vi "Simultaneous Sound Input Output.vi"() -> ()   [LabVIEW 2023]
doc: "This VI illustrates how to perform simultaneous sound IO, i.e., how to continuously play the sound acquired from a microphone. It requires the use of a microphone attached to the sound card. You can specify the IDs of the input and output devices, the frequency to sample at, and the buffer size for both devices. Higher frequencies have better quality, but demand more resources and are limited by the capabilities of your sound card. A large number of samples decreases the risk of glitches, but increases the delay between acquisition and playback."
uses:
  <vilib>/sound2/lvsound2.llb/Sampling Mode.ctl
  <vilib>/sound2/lvsound2.llb/Sound Data Format.ctl
  <vilib>/sound2/lvsound2.llb/Sound Output Write (DBL Single).vi
  <vilib>/sound2/lvsound2.llb/Sound Input Read (DBL).vi
  <vilib>/sound2/lvsound2.llb/Sound Output Write (DBL).vi
panel:
  out "Acquired Sound":waveform(dbl)[](graph)
  in  "Stop":bool
  in  "Input Device ID":u32
  in  "Output Device ID":u32
  # "Overview: Demonstrates the use of the Sound Functions to continuously play the sound acquired from a microphone.\nRequirements: Microphone\nInstructions:\n1. Specify the Input Device ID and the Output Device ID.\n2. Run the VI.\n3. Click Stop to stop the VI."
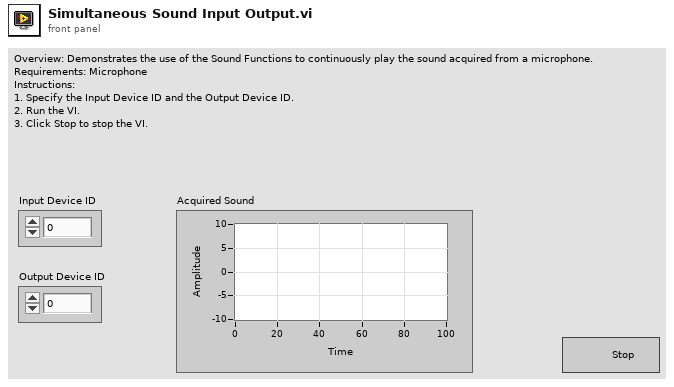
[diagram p1: front panel]
types:
  T1 = typedef "Sound Data Format.ctl" = cluster{"sample rate (S/s)":dbl, "number of channels":i32, "bits per sample":i32}
  T2 = typedef "Sampling Mode.ctl" = i32
  T3 = typedef "Sound Output Task ID.ctl" = u32
  T4 = typedef "Sound Input Task ID.ctl" = u32
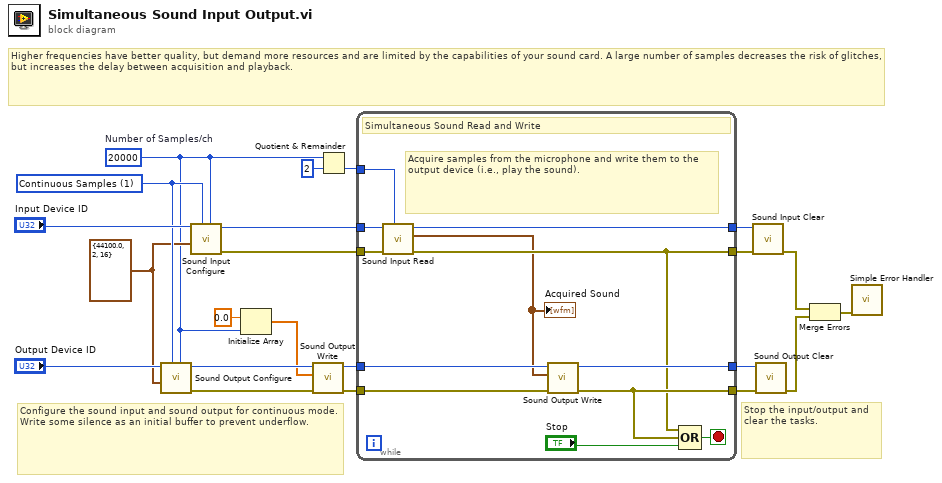
[diagram p0: block diagram]
diagram:
  w2 = 20000  # Number of Samples/ch
  w6 = T1 {"sample rate (S/s)"=44100.0, "number of channels"=2, "bits per sample"=16} ("Sound Format")
  w12 = T2 1 items=["Finite Samples", "Continuous Samples"] ("sample mode")
  # "Higher frequencies have better quality, but demand more resources and are limited by the capabilities of your sound card. A large number of samples decreases the risk of glitches, but increases the delay between acquisition and playback."
  # "Stop the input/output and clear the tasks."
  # "Configure the sound input and sound output for continuous mode. Write some silence as an initial buffer to prevent underflow."
  n1 = call <vilib>:"Sound Output Configure.vi"("number of samples/ch"=w2, "sample mode"=w12, "sound format"=w6, "device ID"="Output Device ID") -> ("error out"=w10:errorcluster, "task ID"=w11:T3)  [unwired: 6 in]
  n2 = call <vilib>:"Sound Input Configure.vi"("number of samples/ch"=w2, "sample mode"=w12, "sound format"=w6, "device ID"="Input Device ID") -> ("error out"=w14:errorcluster, "task ID"=w13:T4)  [unwired: 6 in]
  n3 = Initialize Array(0.0 ("element"), w2) -> (w4:dbl[])
  n4 = call-poly <vilib>:"Sound Output Write.vi"("error in (no error)"=w10, "data"=w4, "task ID"=w11) -> ("error out"=w9:errorcluster, "task ID out"=w8:T3)  [unwired: 7 in]
  n5 = Quotient & Remainder(x=w2, y=2) -> (floor(x/y)=w3:i32)  [unwired: 1 out]
  n6 = while {
    tunnel: w3 -> [w30]
    tunnel: w13 -> [w32]
    tunnel: [w29] -> w17
    tunnel: w8 -> [w33]
    tunnel: [w31] -> w20
    tunnel: w9 -> [w28]
    tunnel: [w25] -> w21
    tunnel: w14 -> [w34]
    tunnel: [w24] -> w22
    stop <- w26 stop-if-true
    # "Acquire samples from the microphone and write them to the output device (i.e., play the sound)."
    # "Simultaneous Sound Read and Write"
    n7 = call-poly <vilib>:"Sound Input Read.vi"("number of samples/ch"=w30, "error in (no error)"=w34, "task ID"=w32) -> ("error out"=w24:errorcluster, "data"=w23:waveform(dbl)[], "task ID out"=w29:T4)  [unwired: 6 in]
    "Acquired Sound" <- w23
    n8 = call-poly <vilib>:"Sound Output Write.vi"("error in (no error)"=w28, "data"=w23, "task ID"=w33) -> ("error out"=w25:errorcluster, "task ID out"=w31:T3)  [unwired: 7 in]
    n9 = Compound Arithmetic op=OR(w24, w25, "Stop") -> (w26:bool)
  }
  n10 = call <vilib>:"Sound Input Clear.vi"("error in (no error)"=w22, "task ID"=w17) -> ("error out"=w15:errorcluster)  [unwired: 9 in]
  n11 = call <vilib>:"Sound Output Clear.vi"("error in (no error)"=w21, "task ID"=w20) -> ("error out"=w16:errorcluster)  [unwired: 9 in]
  n12 = Merge Errors(w15, w16) -> (w7:errorcluster)
  n13 = call <vilib>:"Simple Error Handler.vi"("error in (no error)"=w7) -> ()  [unwired: 4 in, 5 out]
